vi "Create Block.vi"(8 "error in (no error)":errorcluster, 9 "Value":u32, 10 "Available Indexes":cluster{i32, i32}, 11 "Grid":refnum<data-value>) -> (0 "error out":errorcluster, 3 "New Block":refnum<data-value>)   [LabVIEW 2016, in "Block.lvclass"]
uses:
  Block/Block.lvclass
  <vilib>/LIEF/Forms/Shape/Shape.lvclass
  C:/Users/frmausse/Desktop/LIEF Intro Package/LIEF 2048/Gradient Rectangle/Gradient Rectangle.lvclass
  C:/Program Files (x86)/National Instruments/LabVIEW 2016/vi.lib/LIEF/Forms/Shape/Shape.lvclass
  C:/Program Files (x86)/National Instruments/LabVIEW 2016/vi.lib/LIEF/Forms/Layered Shape/Layered Shape.lvclass
  <vilib>/LIEF/Forms/Layered Shape/Layered Shape.lvclass/Layered Shape.ctl
  <vilib>/LIEF/Forms/Layered Shape/Write Overlays.vi
  <vilib>/LIEF/Forms/Text/Text.lvclass
  <vilib>/LIEF/Forms/Grid/Grid.lvclass
  Gradient Rectangle/Gradient Rectangle.lvclass
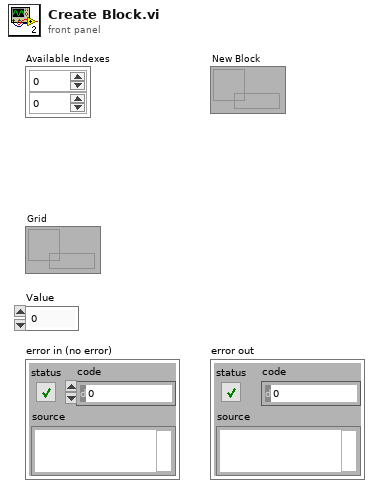
[diagram p1: front panel]
types:
  T1 = cluster{"Font Name:":string, "Size":i16, "Strikeout?":bool, "Italic?":bool, "Underline?":bool, "Outline?":bool, "Shadow?":bool, "Bold?":bool}
  T2 = enum16{"Left", "Top", "Right", "Bottom", "Centered"}
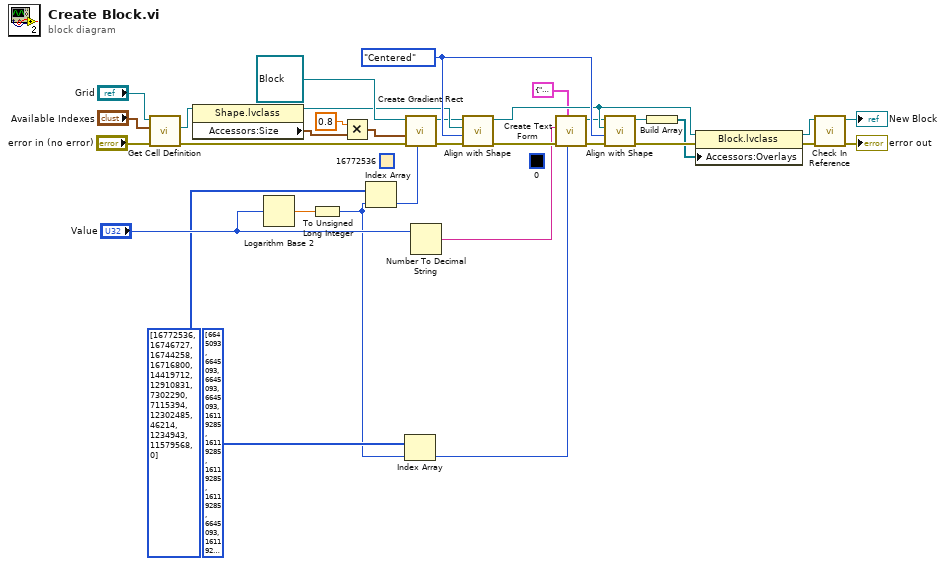
[diagram p0: block diagram]
diagram:
  (unwired) u32 16772536 ("Color")
  (unwired) u32 0 ("Color")
  w19 = T2."Centered" ("Alignment")
  n1 = call <vilib>:"Get Cell Definition.vi"("error in (no error)"="error in (no error)", "Indexes"="Available Indexes", "Shape Reference"="Grid") -> ("error out"=w23:errorcluster, "Cell"=w11:refnum<class "Shape.lvclass">)  [unwired: 6 in, 1 out]
  n2 = property class="Shape.lvclass"(reference=w11) -> (reference out=w14:refnum<class "Shape.lvclass">, "Accessors:Size"=w32:cluster{"Width":i32, "Height":i32})  [unwired: 1 in, 1 out]
  n3 = Logarithm Base 2(1:"Value") -> (0:w7:dbl)
  n4 = To Unsigned Long Integer(number=w7) -> (unsigned 32bit integer=w1:u32)
  n5 = Multiply(x=0.8, y=w32) -> (x*y=w33:cluster{"Width":dbl, "Height":dbl})
  n6 = Index Array(array=u32[] [16772536, 16746727, 16744258, 16716800, 14419712, 12910831, 7302290, 7115394, 12302485, 46214, 1234943, 11579568, 0] ("Color"), index=w1) -> (element=w5:u32)
  n7 = Index Array(array=u32[] [6645093, 6645093, 6645093, 6645093, 16119285, 16119285, 16119285, 16119285, 6645093, 16119285, 6645093, 6645093, 16119285] ("Color"), index=w1) -> (element=w3:u32)
  n8 = call "Create Gradient Rect.vi"("Color"=w5, "error in (no error)"=w23, "Size"=w33, "Gradient Rectangle in"=refnum<class "Block.lvclass"> refnum ("Block in")) -> ("error out"=w12:errorcluster, "Gradient Rectangle out"=w13:refnum<class "Block.lvclass">)  [unwired: 6 in]
  n9 = Number To Decimal String(number="Value") -> (decimal integer string=w9:string)  [unwired: 1 in]
  n10 = call <vilib>:"Align with Shape.vi"("error in (no error)"=w12, "Alignment"=w19, "Reference Shape"=w14, "Shape in"=w13) -> ("error out"=w25:errorcluster, "Shape out"=w17:refnum<class "Block.lvclass">)  [unwired: 6 in]
  n11 = call <vilib>:"Create Text Form.vi"("Color"=w3, "[user-specified font]"=T1 {"Font Name:"="Verdana", "Size"=28, "Strikeout?"=FALSE, "Italic?"=FALSE, "Underline?"=FALSE, "Outline?"=FALSE, "Shadow?"=FALSE, "Bold?"=TRUE}, "error in (no error)"=w25, "Text"=w9) -> ("error out"=w15:errorcluster, "New Text"=w16:refnum<class "Text.lvclass">)  [unwired: 6 in]
  n12 = call <vilib>:"Align with Shape.vi"("error in (no error)"=w15, "Alignment"=w19, "Reference Shape"=w17, "Shape in"=w16) -> ("error out"=w24:errorcluster, "Shape out"=w18:refnum<class "Text.lvclass">)  [unwired: 6 in]
  n13 = Build Array(w18) -> (w20:refnum<class "Text.lvclass">[])
  n14 = property class="Block.lvclass"(reference=w17, error in=w24, "Accessors:Overlays"=w20) -> (reference out=w21:refnum<class "Block.lvclass">, error out=w26:errorcluster)
  n15 = call <vilib>:"Check In Reference.vi"("error in (no error)"=w26, "Shape in"=w21) -> ("error out"=→"error out":errorcluster, "Shape Reference"=→"New Block":refnum<data-value>)  [unwired: 8 in]
